vi "Initialise.vi"(6 "Tag Root":string, 8 "error in (no error)":errorcluster, 10 "FPGA Interface":refnum<k20>, 11 "FPGA-Bus in":refnum<class "FPGA-Bus.lvclass">) -> (0 "error out":errorcluster, 3 "FPGA-Bus out":refnum<class "FPGA-Bus.lvclass">)   [LabVIEW 2021, in "FPGA-Bus.lvclass"]
uses:
  FPGA-Bus.lvclass
  C:/Program Files (x86)/National Instruments/LabVIEW 2021/vi.lib/TSA/Omni-Bus/Omni-Bus/Bus Access/Bus_Access.lvclass
  FPGA-Bus.lvclass/FPGA-Bus.ctl
  <vilib>/TSA/Omni-Bus/Omni-Bus/Bus Access/Bus_Access.lvclass/Bus_Access.ctl
  Properties/Write FPGA Interface.vi
  <vilib>/TSA/Omni-Bus/Omni-Bus/Bus Access/Properties/Write Tag Root.vi
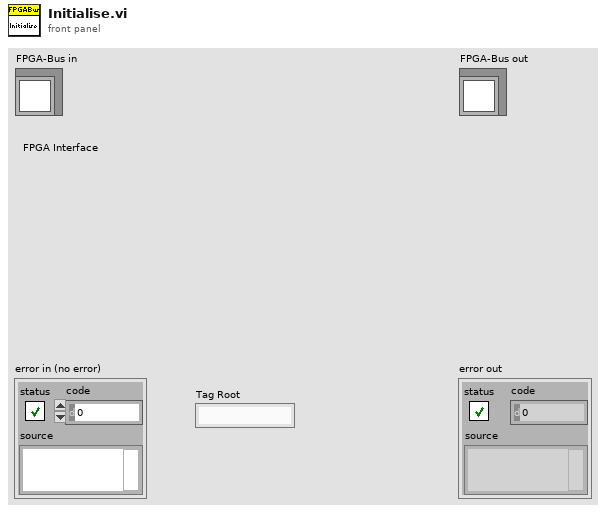
[diagram p1: front panel]
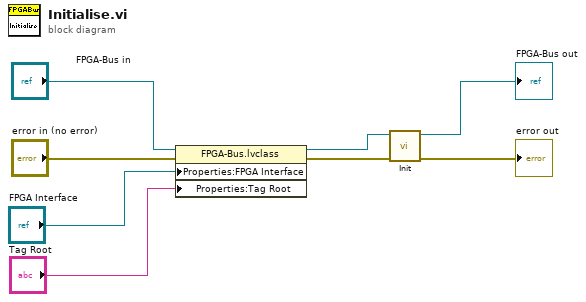
[diagram p0: block diagram]
diagram:
  n1 = property class="FPGA-Bus.lvclass"(reference="FPGA-Bus in", error in="error in (no error)", "Properties:FPGA Interface"="FPGA Interface", "Properties:Tag Root"="Tag Root") -> (reference out=w2:refnum<class "FPGA-Bus.lvclass">, error out=w3:errorcluster)
  n2 = call-dynamic "Init.vi"("error in (no error)"=w3, "Data in"=w2) -> ("error out"=→"error out":errorcluster, "Data out"=→"FPGA-Bus out":refnum<class "FPGA-Bus.lvclass">)  [unwired: 8 in]
